vi "Input_Dashboard_Commands.vi"(11 "All Joysticks":T2) -> (3 "Dashboard Controls":T1)   [LabVIEW 2012]
uses:
  Input_All_Joysticks.ctl
  Input_Single_Joystick.ctl
  <vilib>/Rock Robotics/WPI/Joystick/WPI_JoystickButtonState.ctl
  Dashboard Controls.ctl
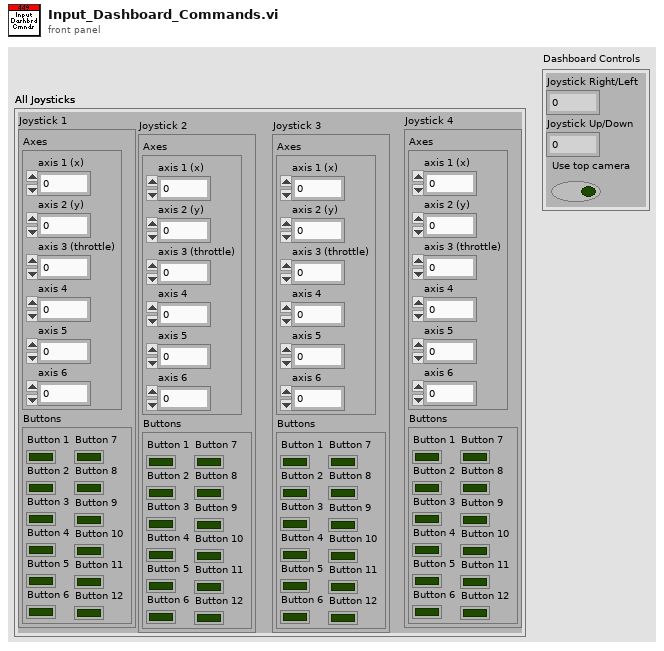
[diagram p1: front panel]
types:
  T1 = typedef "Dashboard Controls.ctl" = cluster{"Joystick Right/Left":dbl, "Joystick Up/Down":dbl, "Use top camera":bool}
  T2 = typedef "Input_All_Joysticks.ctl" = cluster{"Joystick 1":T3, "Joystick 2":T3, "Joystick 3":T3, "Joystick 4":T3}
  T3 = typedef "Input_Single_Joystick.ctl" = cluster{"Axes":cluster{"axis 1 (x)":dbl, "axis 2 (y)":dbl, "axis 3 (throttle)":dbl, "axis 4":dbl, "axis 5":dbl, "axis 6":dbl}, "Buttons":T4}
  T4 = typedef "WPI_JoystickButtonState.ctl" = cluster{"Button 1":bool, "Button 2":bool, "Button 3":bool, "Button 4":bool, "Button 5":bool, "Button 6":bool, "Button 7":bool, "Button 8":bool, "Button 9":bool, "Button 10":bool, "Button 11":bool, "Button 12":bool}
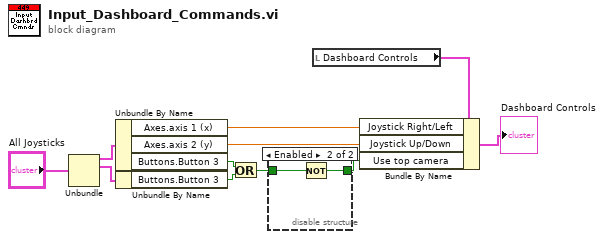
[diagram p0: block diagram]
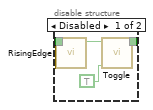
[diagram p2: hidden frame]
diagram:
  n1 = Unbundle("All Joysticks") -> ("Joystick 1"=w8:T3, "Joystick 2"=w5:T3)  [unwired: 2 out]
  n2 = Unbundle By Name(w8) -> ("Axes.axis 1 (x)"=w7:dbl, "Axes.axis 2 (y)"=w6:dbl, "Buttons.Button 3"=w4:bool)
  n3 = Unbundle By Name(w5) -> ("Buttons.Button 3"=w3:bool)
  n4 = Or(x=w4, y=w3) -> (x .or. y?=w2:bool)
  n5 = disable-structure shown="Enabled" {
    disable-tunnel: w2 -> [w15 w17]
    disable-tunnel: [w14 w16] -> w1
    frame Disabled {
      n6 = call "RisingEdge.vi"("BooleanIn"=w15) -> ("BooleanOut"=w12:bool)  [unwired: 10 in]
      n7 = call "Toggle.vi"("Initial"=TRUE, "Toggle"=w12) -> ("BoolOut"=w14:bool)  [unwired: 9 in]
    }
    frame Enabled {
      n8 = Not(x=w17) -> (.not. x?=w16:bool)
    }
  }
  n9 = local read "Dashboard Controls"() -> (w10:T1)
  n10 = Bundle By Name(cluster=w10, "Joystick Right/Left"=w7, "Joystick Up/Down"=w6, "Use top camera"=w1) -> (→"Dashboard Controls":T1)
